vi "csv sender.vi"() -> ()   [LabVIEW 2021]
panel:
  in  "Boolean":bool
  in  "loop 1":i32
  out "Numeric 3":dbl
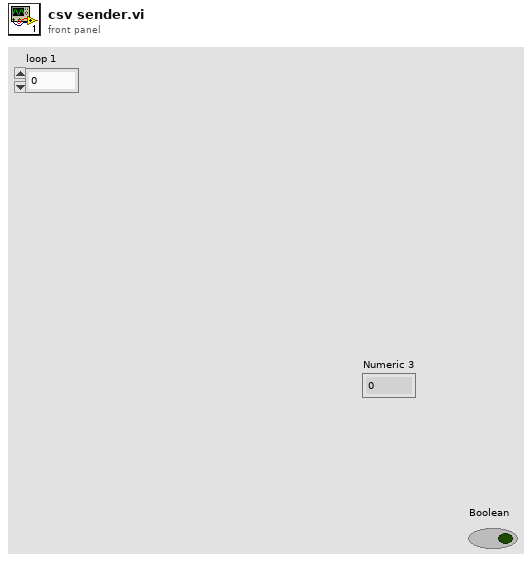
[diagram p1: front panel]
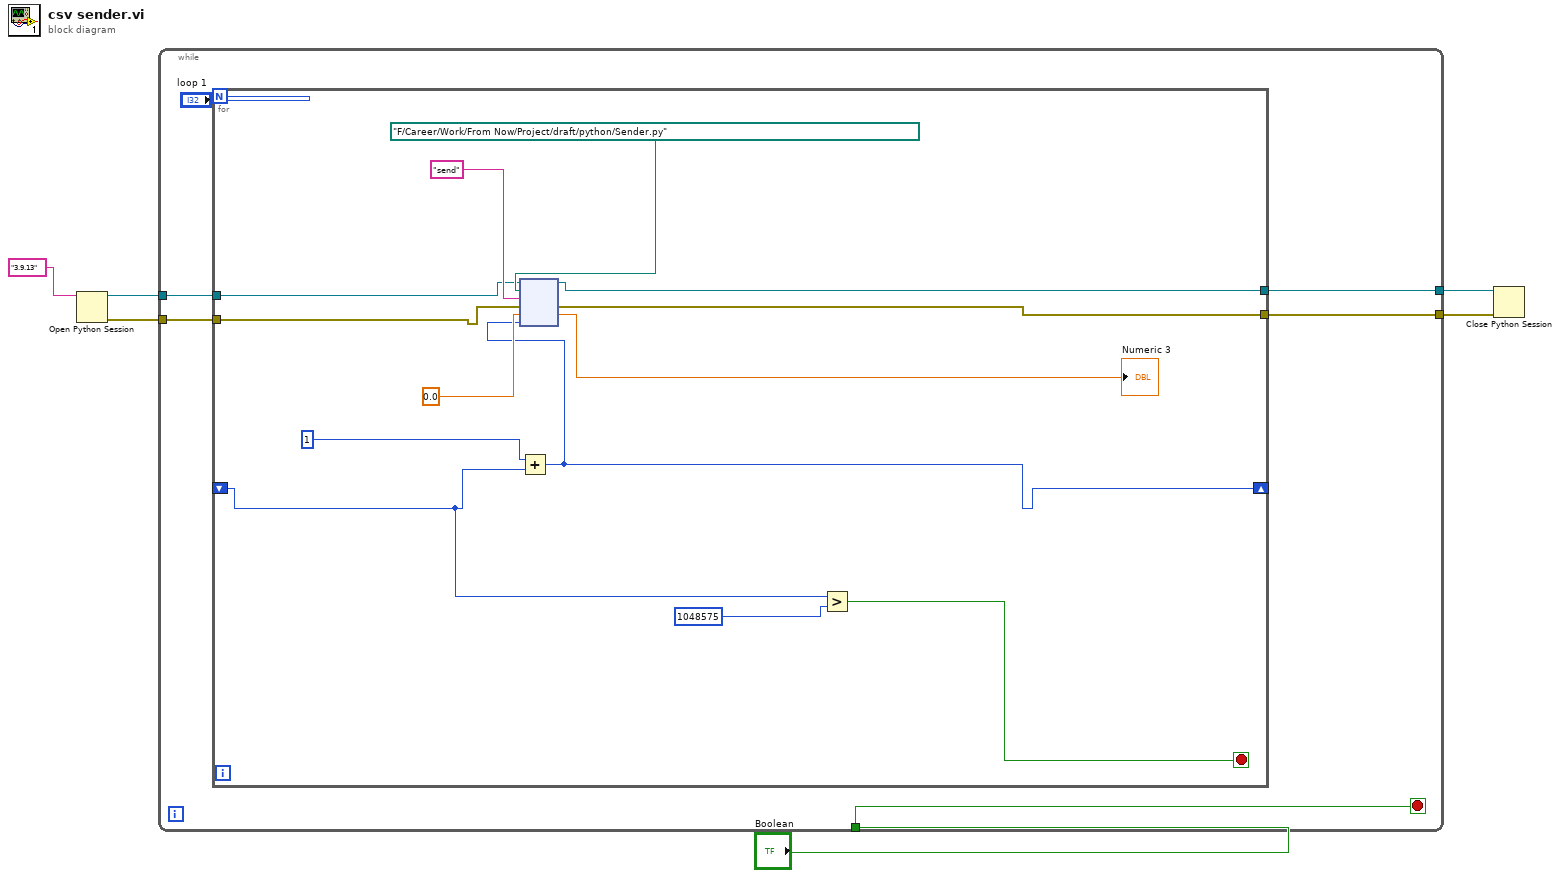
[diagram p0: block diagram]
diagram:
  n1 = Open Python Session(python version="3.9.13" ("Python version")) -> (session out=w4:refnum<k35>, error out=w3:errorcluster)  [unwired: 2 in]
  n2 = while {
    tunnel: "Boolean" -> [w12]
    tunnel: w4 -> [w10]
    tunnel: w3 -> [w9]
    tunnel: [w8] -> w2
    tunnel: [w7] -> w1
    stop <- w12 stop-if-true
    n3 = for {
      N: "loop 1" -> [_]
      shift-right: [w18] -> _
      shift-left: _ -> [w19]
      tunnel: w10 -> [w16]
      tunnel: w9 -> [w15]
      tunnel: [w14] -> w8
      tunnel: [w13] -> w7
      stop <- w17 stop-if-true
      n4 = Add(x=1, y=w19) -> (x+y=w18:i32)
      n5 = node(w16, path "F:/Career/Work/From Now/Project/draft/python/Sender.py" ("module path"), "send" ("function name"), w15, 0.0, w18) -> (w14:refnum<k35>, w13:errorcluster, →"Numeric 3":dbl)  [unwired: 1 in, 2 out]
      n6 = Greater?(x=w19, y=1048575) -> (0:w17:bool)
    }
  }
  n7 = Close Python Session(session in=w2, error in=w1) -> ()  [unwired: 1 out]
